vi "Print.vi"(8 "error in (no error)":errorcluster, 11 "Pizza(Product) in":refnum<class "Pizza(Product).lvclass">) -> (0 "error out":errorcluster, 3 "Pizza(Product) out":refnum<class "Pizza(Product).lvclass">)   [LabVIEW 2014, in "Pizza(Product).lvclass"]
uses:
  Pizza(Product).lvclass
  Pizza(Product).lvclass/Pizza(Product).ctl
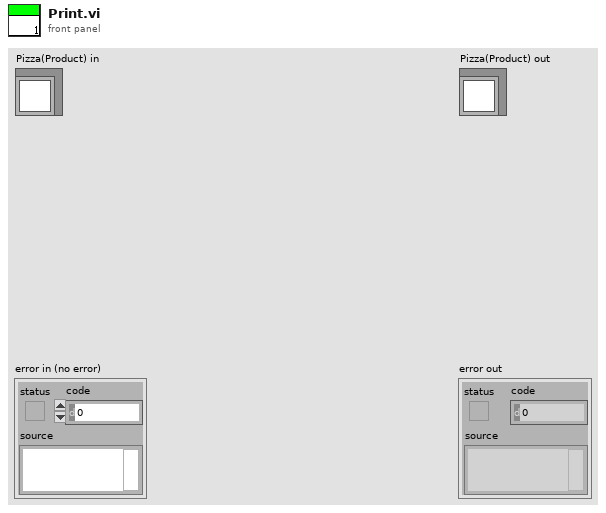
[diagram p1: front panel]
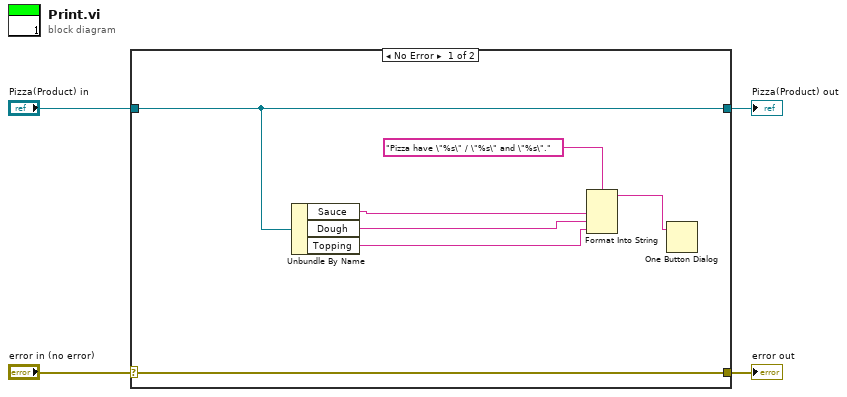
[diagram p0: block diagram]
diagram:
  n1 = case shown="No Error" "error in (no error)" {
    selector: "error in (no error)" -> [w11 w13]
    tunnel: [w11 w13] -> w3
    tunnel: [w5 w12] -> w1
    tunnel: "Pizza(Product) in" -> [w5 w12]
    frame No Error {
      n2 = Unbundle By Name(w5) -> ("Sauce"=w6:string, "Dough"=w10:string, "Topping"=w9:string)
      n3 = Format Into String(format string="Pizza have \"%s\" / \"%s\" and \"%s\".", w6, w10, w9) -> (resulting string=w7:string)  [unwired: 2 in, 1 out]
      n4 = One Button Dialog(message=w7) -> ()  [unwired: 1 in, 1 out]
    }
    frame Error {
    }
  }
  "error out" <- w3
  "Pizza(Product) out" <- w1
